vi "ramp.vi"(0 "Log Scale?":bool, 1 "Array":dbl[][](array[numeric]), 2 "Instrument Address":refnum<visa-resource-name>) -> ()   [LabVIEW 2020]
panel:
  out "Time Remaining":dbl format="%<%H:%M:%S>t"
  out "Status Line":string
  in  "Pause":bool
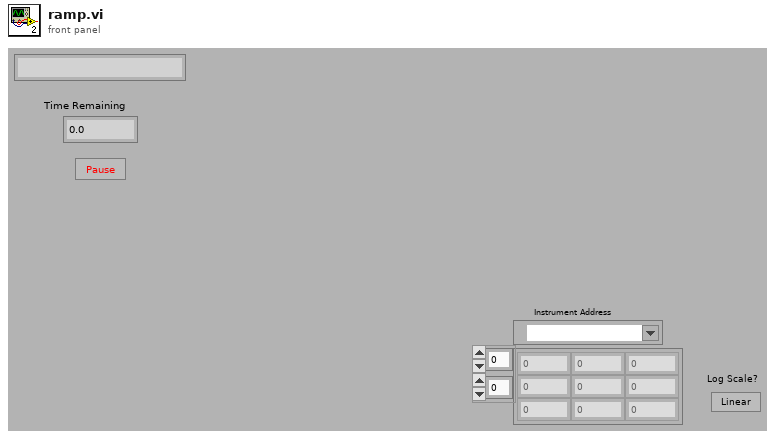
[diagram p1: front panel]
types:
  T1 = cluster{"Setpoint":dbl, "Ramp Time":dbl, "Soak Time":dbl}
  T2 = cluster{"Array[0]":dbl, "Array[1]":dbl, "Array[2]":dbl}
  T3 = enum16{"Left Button", "Center Button", "Right Button", "Window Close"}
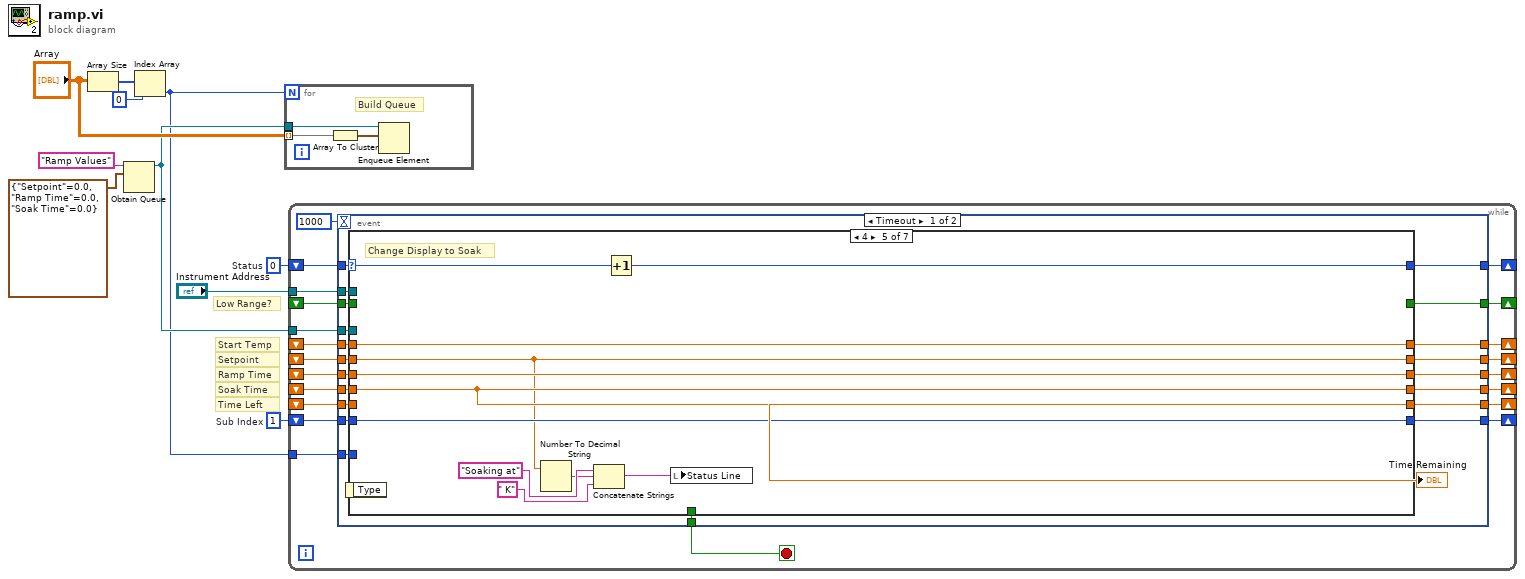
[diagram p0: block diagram]
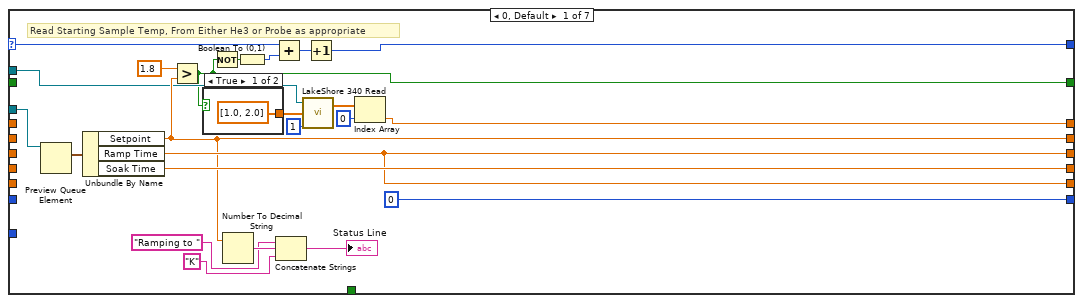
[diagram p2: hidden frame]
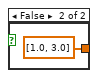
[diagram p3: hidden frame]
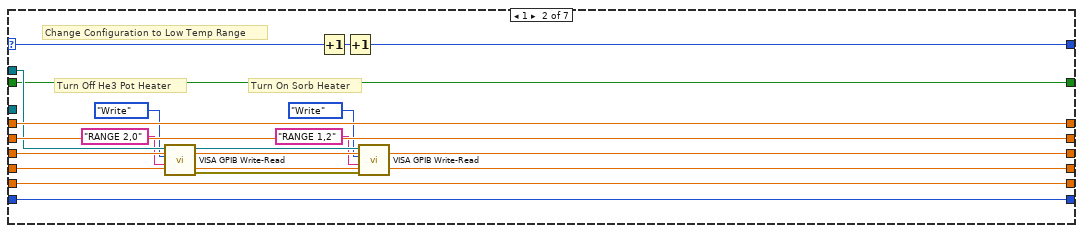
[diagram p4: hidden frame]
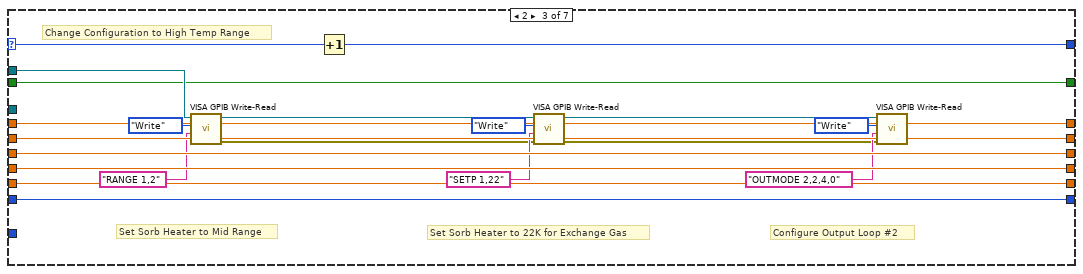
[diagram p5: hidden frame]
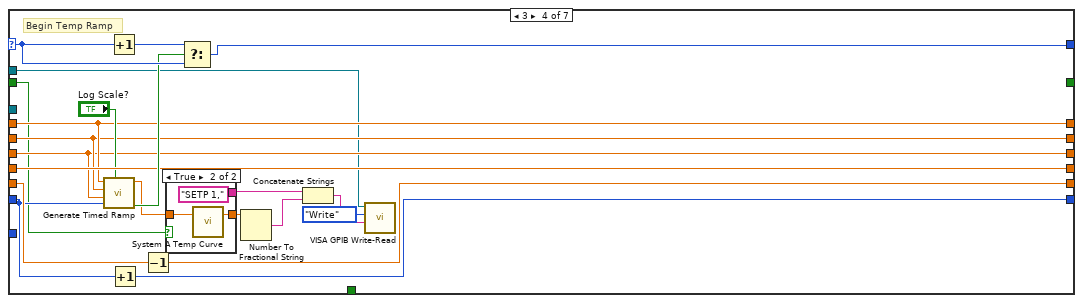
[diagram p6: hidden frame]
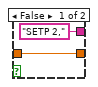
[diagram p7: hidden frame]
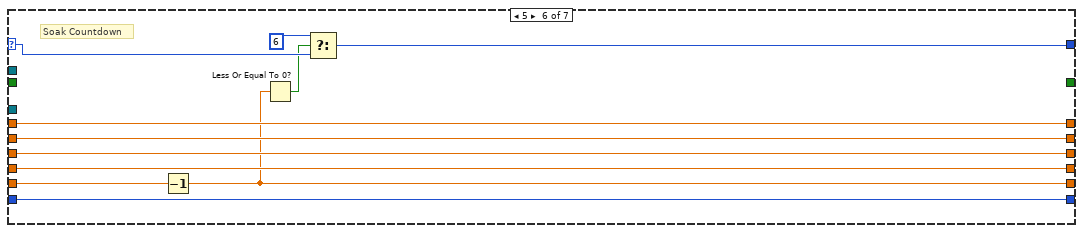
[diagram p8: hidden frame]
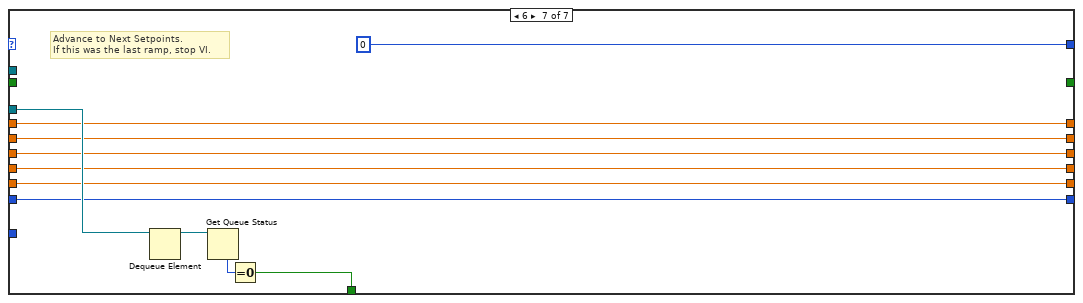
[diagram p9: hidden frame]
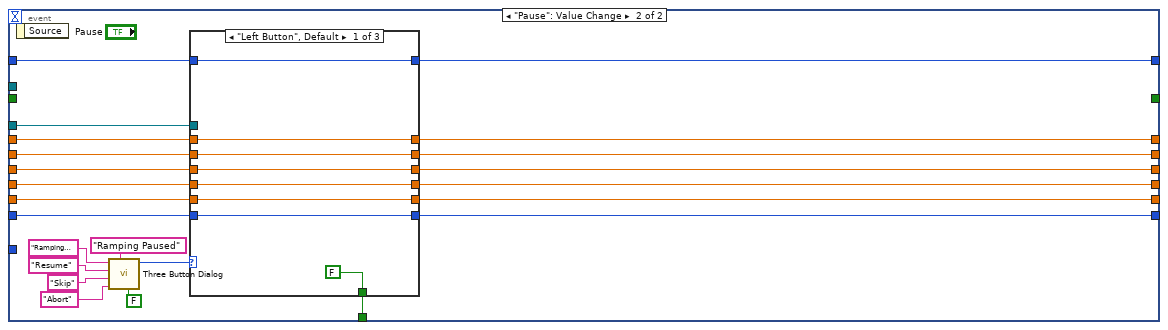
[diagram p10: hidden frame]
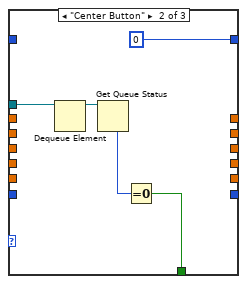
[diagram p11: hidden frame]
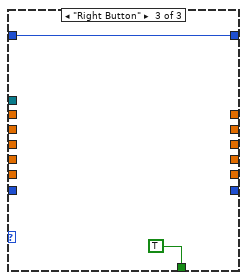
[diagram p12: hidden frame]
diagram:
  w2 = 1  # Sub Index
  w5 = 0  # Status
  # "Low Range?"
  # "Time Left"
  # "Start Temp"
  # "Soak Time"
  # "Ramp Time"
  # "Setpoint"
  n1 = Array Size(array="Array") -> (size(s)=w8:i32[])
  n2 = Obtain Queue(name (unnamed)="Ramp Values", element data type=T1 {"Setpoint"=0.0, "Ramp Time"=0.0, "Soak Time"=0.0}) -> (queue out=w3:refnum<queue>)  [unwired: 3 in, 2 out]
  n3 = Index Array(array=w8, index=0) -> (element=w1:i32)
  n4 = for {
    N: w1 -> [_]
    tunnel: "Array" -> [w13] mode=indexing
    tunnel: w3 -> [w12]
    # "Build Queue"
    n5 = Array To Cluster(array=w13) -> (cluster=w11:T2)
    n6 = Enqueue Element(queue=w12, element=w11) -> ()  [unwired: 2 in, 3 out]
  }
  n7 = while {
    tunnel: "Instrument Address" -> [w32]
    tunnel: w3 -> [w31]
    shift-right: [w30] -> _
    shift-left: _ -> [w26]
    shift-right: [w29] -> _
    shift-left: _ -> [w25]
    shift-right: [w28] -> _
    shift-left: _ -> [w24]
    shift-right: [w27] -> _
    shift-left: w5 -> [w33]
    shift-right: [w23] -> _
    shift-left: _ -> [w22]
    shift-right: [w18] -> _
    shift-left: w2 -> [w21]
    shift-right: [w20] -> _
    shift-left: _ -> [w19]
    tunnel: w1 -> [w16]
    shift-right: [w15] -> _
    shift-left: _ -> [w14]
    stop <- w17 stop-if-true
    n8 = event shown="[0] Timeout" {
      selector: _ -> [_ _]
      dyn-events: _ -> [_ _]
      timeout: 1000 -> [_ _]
      tunnel: w33 -> [w54 w189]
      tunnel: w32 -> [w53 _]
      tunnel: w31 -> [w52 w192]
      tunnel: [w40 w185] -> w30
      tunnel: [w51 w183] -> w29
      tunnel: [w50 w181] -> w28
      tunnel: [w41 w191] -> w27
      tunnel: w26 -> [w48 w186]
      tunnel: w25 -> [w47 w184]
      tunnel: w24 -> [w46 w182]
      tunnel: [w39 w187] -> w23
      tunnel: w22 -> [w49 w188]
      tunnel: w21 -> [w45 w178]
      tunnel: [w37 w179] -> w20
      tunnel: w19 -> [w44 w180]
      tunnel: [w43 w177] -> w18
      tunnel: [w42 w190] -> w17
      tunnel: w16 -> [w38 _]
      tunnel: [w36 _] -> w15
      tunnel: w14 -> [w35 _]
      event Timeout {
        n9 = event-data() -> ()  [unwired: 1 in, 1 out]
        n10 = case shown="4" w54 {
          selector: w54 -> [w58 w91 w111 w137 w153 w158 _]
          tunnel: w53 -> [w61 w88 w109 w123 _ _ _]
          tunnel: w52 -> [w73 _ _ _ _ _ w174]
          tunnel: [w62 w89 w110 w125 w146 w163 w166] -> w40
          tunnel: [w70 w95 w115 w124 w151 w162 w167] -> w51
          tunnel: [w71 w94 w114 w129 w150 w161 w168] -> w50
          tunnel: [w55 w87 w108 w134 w148 w159 0] -> w41
          tunnel: [w64 w96 w116 w126 w152 w164 w165] -> w39
          tunnel: w49 -> [_ w96 w116 w126 w152 w164 w165]
          tunnel: w48 -> [_ w89 w110 w125 w146 w163 w166]
          tunnel: w47 -> [_ w95 w115 w124 w151 w162 w167]
          tunnel: w46 -> [_ w94 w114 w129 w150 w161 w168]
          tunnel: w45 -> [_ w92 w112 w120 w149 w154 w170]
          tunnel: [w70 w93 w113 w121 w150 w156 w169] -> w37
          tunnel: w44 -> [_ w93 w113 w122 _ w160 w169]
          tunnel: [0 w92 w112 w119 w149 w154 w170] -> w43
          tunnel: [_ _ _ _ _ _ w171] -> w42
          tunnel: w38 -> [_ _ _ _ _ _ _]
          tunnel: [w57 w86 w107 _ _ _ _] -> w36
          tunnel: w35 -> [_ w86 w107 w118 _ _ _]
          frame 0, Default {
            # "Read Starting Sample Temp, From Either He3 or Probe as appropriate"
            n11 = Preview Queue Element(queue=w73) -> (element=w72:T1)  [unwired: 2 in, 3 out]
            n12 = Unbundle By Name(w72) -> ("Setpoint"=w62:dbl, "Ramp Time"=w70:dbl, "Soak Time"=w71:dbl)
            n13 = Greater?(x=1.8, y=w62) -> (0:w57:bool)
            n14 = case shown="True" w57 {
              tunnel: [dbl[] [1.0, 2.0] ("Parameters") dbl[] [1.0, 3.0] ("Parameters")] -> w74
              frame True {
              }
              frame False {
              }
            }
            n15 = Not(x=w57) -> (.not. x?=w56:bool)
            n16 = Number To Decimal String(number=w62) -> (decimal integer string=w67:string)  [unwired: 1 in]
            n17 = Boolean To (0,1)(Boolean=w56) -> (0, 1=w60:i16)
            n18 = Add(x=w58, y=w60) -> (x+y=w59:i32)
            n19 = Concatenate Strings("Ramping to " ("string"), w67, "K" ("string")) -> (→"Status Line":string)
            n20 = call "LakeShore 340 Read.vi"("Point #"=1, "Parameters"=w74, "Instrument Address"=w61) -> ("Measurement"=w76:dbl[])  [unwired: 1 out]
            n21 = Increment(x=w59) -> (x+1=w55:i32)
            n22 = Index Array(array=w76, index=0) -> (element=w64:dbl)
          }
          frame 1 {
            # "Turn On Sorb Heater"
            # "Turn Off He3 Pot Heater"
            # "Change Configuration to Low Temp Range"
            n23 = call "VISA GPIB Write-Read.vi"("Command"="RANGE 2,0" ("Command String"), "Action"=enum16{"Write", "Read", "Write & Read"}."Write", "VISA resource name"=w88) -> ("error out"=w80:errorcluster, "dup VISA Session"=w85:refnum<visa-resource-name>)  [unwired: 5 in, 2 out]
            n24 = Increment(x=w91) -> (x+1=w90:i32)
            n25 = Increment(x=w90) -> (x+1=w87:i32)
            n26 = call "VISA GPIB Write-Read.vi"("error in (no error)"=w80, "Command"="RANGE 1,2" ("Command String"), "Action"=enum16{"Write", "Read", "Write & Read"}."Write", "VISA resource name"=w85) -> ()  [unwired: 4 in, 4 out]
          }
          frame 2 {
            # "Set Sorb Heater to 22K for Exchange Gas"
            # "Configure Output Loop #2"
            # "Set Sorb Heater to Mid Range"
            # "Change Configuration to High Temp Range"
            n27 = call "VISA GPIB Write-Read.vi"("Command"="RANGE 1,2" ("Command String"), "Action"=enum16{"Write", "Read", "Write & Read"}."Write", "VISA resource name"=w109) -> ("error out"=w100:errorcluster, "dup VISA Session"=w106:refnum<visa-resource-name>)  [unwired: 5 in, 2 out]
            n28 = Increment(x=w111) -> (x+1=w108:i32)
            n29 = call "VISA GPIB Write-Read.vi"("error in (no error)"=w100, "Command"="SETP 1,22" ("Command String"), "Action"=enum16{"Write", "Read", "Write & Read"}."Write", "VISA resource name"=w106) -> ("error out"=w99:errorcluster, "dup VISA Session"=w103:refnum<visa-resource-name>)  [unwired: 4 in, 2 out]
            n30 = call "VISA GPIB Write-Read.vi"("error in (no error)"=w99, "Command"="OUTMODE 2,2,4,0" ("Command String"), "Action"=enum16{"Write", "Read", "Write & Read"}."Write", "VISA resource name"=w103) -> ()  [unwired: 4 in, 4 out]
          }
          frame 3 {
            # "Begin Temp Ramp"
            n31 = call "Generate Timed Ramp.vi"("Log"="Log Scale?", "Point #"=w120, "Time (Hr:Min:Sec)"=w124, "Stop"=w125, "Start"=w126) -> ("Stop"=w135:bool, "Output"=w128:dbl)  [unwired: 2 out]
            n32 = Increment(x=w137) -> (x+1=w136:i32)
            n33 = Increment(x=w120) -> (x+1=w119:i32)
            n34 = Decrement(x=w122) -> (x-1=w121:dbl)
            n35 = case shown="True" w118 {
              tunnel: ["SETP 2," ("String to Write") "SETP 1," ("String to Write")] -> w132
              tunnel: [w139 w141] -> w130
              tunnel: w128 -> [w139 w140]
              frame False {
              }
              frame True {
                n36 = call "System A Temp Curve.vi"("He3 Goal Temp"=w140) -> ("Corresponding Sorb Temp"=w141:dbl)  [unwired: 1 in, 1 out]
              }
            }
            n37 = Select(t=w136, s=w135, f=w137) -> (s? t:f=w134:i32)
            n38 = Number To Fractional String(number=w130) -> (F-format string=w133:string)  [unwired: 3 in]
            n39 = Concatenate Strings(w132, w133) -> (w131:string)
            n40 = call "VISA GPIB Write-Read.vi"("Command"=w131, "Action"=enum16{"Write", "Read", "Write & Read"}."Write", "VISA resource name"=w123) -> ()  [unwired: 5 in, 4 out]
          }
          frame 4 {
            # "Change Display to Soak"
            n41 = Number To Decimal String(number=w146) -> (decimal integer string=w143:string)  [unwired: 1 in]
            n42 = Concatenate Strings("Soaking at" ("string"), w143, " K" ("string")) -> (w147:string)
            n43 = Increment(x=w153) -> (x+1=w148:i32)
            n44 = local write "Status Line"(w147) -> ()
          }
          frame 5 {
            # "Soak Countdown"
            n45 = Decrement(x=w160) -> (x-1=w156:dbl)
            n46 = Less Or Equal To 0?(x=w156) -> (x <= 0?=w155:bool)
            n47 = Select(t=6, s=w155, f=w158) -> (s? t:f=w159:i32)
          }
          frame 6 {
            # "Advance to Next Setpoints.\nIf this was the last ramp, stop VI."
            n48 = Dequeue Element(queue=w174) -> (queue out=w173:refnum<queue>)  [unwired: 2 in, 3 out]
            n49 = Get Queue Status(queue=w173) -> (# elements in queue=w172:i32)  [unwired: 2 in, 7 out]
            n50 = Equal To 0?(x=w172) -> (x = 0?=w171:bool)
          }
        }
        "Time Remaining" <- w37
      }
      event "Pause": Value Change {
        n51 = event-data() -> ()  [unwired: 1 in, 1 out]
        n52 = call <vilib>:"Three Button Dialog.vi"("Allow user to close window? (TRUE)"=FALSE, "Window Title (\"\")"="Ramping Paused" ("Window Title (\"\")"), "Right Button Text (\"Cancel\")"="Abort" ("Right Button Text (\"Cancel\")"), "Center Button Text (\"No\")"="Skip" ("Center Button Text (\"No\")"), "Left Button Text (\"Yes\")"="Resume" ("Left Button Text (\"Yes\")"), "message"="Ramping has been paused.  Do you wish to: \nResume where you left off, \nSkip this setpoint and procede to the next, or \nAbort all ramping?") -> ("Which Button?"=w193:T3)  [unwired: 5 in]
        n53 = case shown="\"Left Button\", Default" w193 {
          tunnel: w192 -> [_ w211 _]
          tunnel: [w206 0 w212] -> w191
          tunnel: [FALSE w207 TRUE] -> w190
          tunnel: w189 -> [w206 _ w212]
          tunnel: [w205 _ _] -> w187
          tunnel: w188 -> [w205 _ _]
          tunnel: [w204 _ _] -> w185
          tunnel: w186 -> [w204 _ _]
          tunnel: [w203 _ _] -> w183
          tunnel: w184 -> [w203 _ _]
          tunnel: [w202 _ _] -> w181
          tunnel: w182 -> [w202 _ _]
          tunnel: [w201 _ _] -> w179
          tunnel: w180 -> [w201 _ _]
          tunnel: w178 -> [w200 _ _]
          tunnel: [w200 _ _] -> w177
          frame "Left Button", Default {
          }
          frame "Center Button" {
            n54 = Dequeue Element(queue=w211) -> (queue out=w209:refnum<queue>)  [unwired: 2 in, 3 out]
            n55 = Get Queue Status(queue=w209) -> (# elements in queue=w208:i32)  [unwired: 2 in, 7 out]
            n56 = Equal To 0?(x=w208) -> (x = 0?=w207:bool)
          }
          frame "Right Button" {
          }
        }
      }
    }
  }
